vi "simx Get Collection Handle.vi"(7 "operationMode":i32, 8 "error in (no error)":errorcluster, 9 "handle":i32, 10 "collectionName":string, 11 "clientID":i32) -> (0 "error out":errorcluster, 1 "handle out":i32, 3 "function return":i32)   [LabVIEW 2019, in "PXL_V-REP.lvlib"]
doc: "EXTAPI_DLLEXPORT simxInt simxGetCollectionHandle(simxInt clientID,const simxChar* collectionName,simxInt* handle,simxInt operationMode);"
uses:
  PXL_V-REP.lvlib
  <userlib>/V-REP/remoteApi.dll
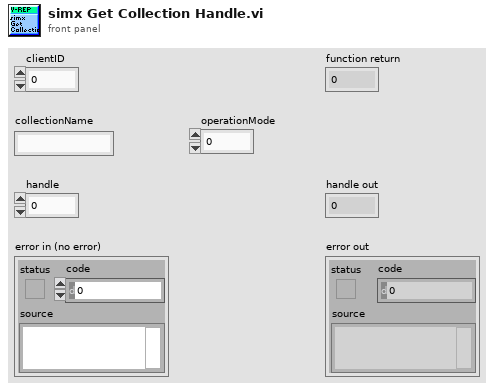
[diagram p1: front panel]
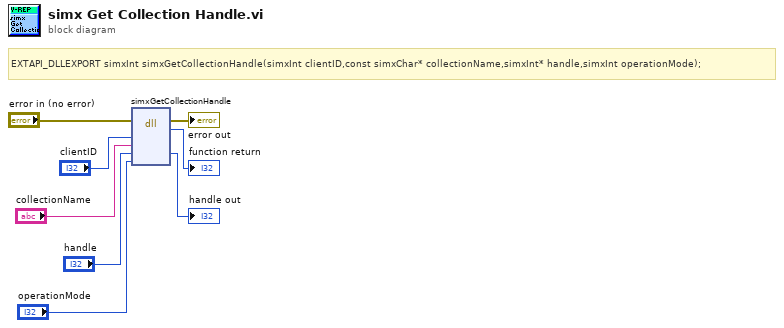
[diagram p0: block diagram]
diagram:
  # "EXTAPI_DLLEXPORT simxInt simxGetCollectionHandle(simxInt clientID,const simxChar* collectionName,simxInt* handle,simxInt operationMode);"
  n1 = dll-call lib="C:/Program Files (x86)/National Instruments/LabVIEW 2019/user.lib/V-REP/remoteApi.*" fn="simxGetCollectionHandle"(error in="error in (no error)", "clientID"="clientID", "collectionName"="collectionName", "handle"="handle", "operationMode"="operationMode") -> (error out=→"error out":errorcluster, →"function return":i32, "handle"=→"handle out":i32)  [unwired: 5 in, 1 out]
